vi "List Controls and Indicators.vi"(8 "error in (no error)":errorcluster, 11 "reference":refnum<vi>) -> (0 "error out":errorcluster, 1 "Controls":refnum<vi>[](array[refnum]), 2 "Indicators":refnum<vi>[](array[refnum]))   [LabVIEW 2017]
panel:
  in  "Array 2":refnum<vi>[](array[refnum])
  in  "Array":refnum<vi>[](array[refnum])
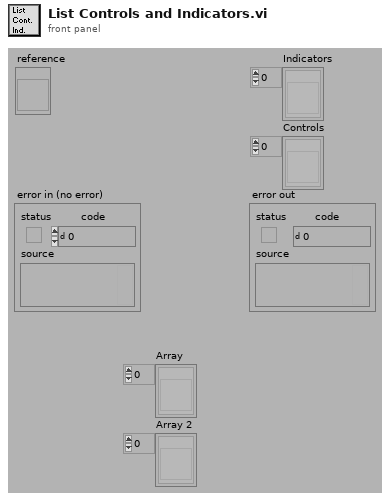
[diagram p1: front panel]
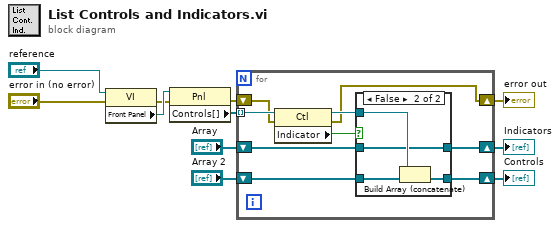
[diagram p0: block diagram]
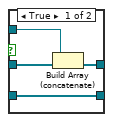
[diagram p2: hidden frame]
diagram:
  n1 = property class="VI"(reference="reference", error in="error in (no error)") -> (error out=w5:errorcluster, "Front Panel"=w11:refnum<vi>)  [unwired: 1 out]
  n2 = property class="Pnl"(reference=w11, error in=w5) -> (error out=w4:errorcluster, "Controls[]"=w10:refnum<vi>[])  [unwired: 1 out]
  n3 = for {
    tunnel: w10 -> [w20] mode=indexing
    shift-right: [w17] -> w7
    shift-left: "Array" -> [w16]
    shift-right: [w14] -> w6
    shift-left: "Array 2" -> [w15]
    shift-right: [w12] -> w3
    shift-left: w4 -> [w13]
    n4 = property class="Ctl"(reference=w20, error in=w13) -> (reference out=w18:refnum<vi>, error out=w12:errorcluster, "Indicator"=w19:bool)
    n5 = case shown="False" w19 {
      tunnel: w18 -> [w24 w26]
      tunnel: [w23 w25] -> w17
      tunnel: w16 -> [w22 w25]
      tunnel: w15 -> [w21 w28]
      tunnel: [w21 w27] -> w14
      frame True {
        n6 = Build Array (concatenate)(w24, w22) -> (w23:refnum<vi>[])
      }
      frame False {
        n7 = Build Array (concatenate)(w26, w28) -> (w27:refnum<vi>[])
      }
    }
  }
  "Indicators" <- w7
  "Controls" <- w6
  "error out" <- w3
